vi "LSMHDR_write.vi"(8 "error in (no error)":errorcluster, 10 "LSMHDR":T1, 11 "refnum in":refnum<file>) -> (0 "error out":errorcluster, 3 "refnum out":refnum<file>)   [LabVIEW 2012]
uses:
  TTTR_data_headers/LSMHDR.ctl
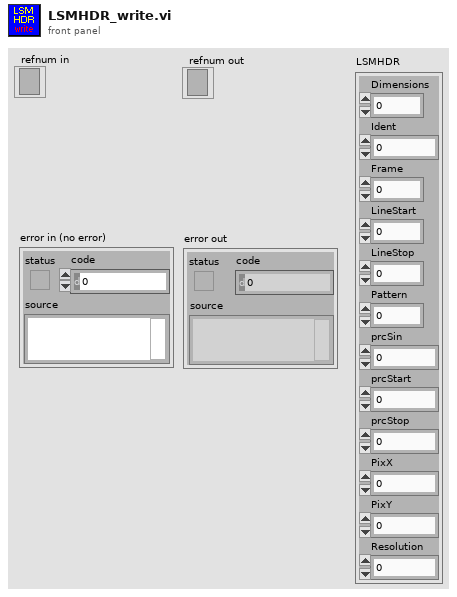
[diagram p1: front panel]
types:
  T1 = typedef "LSMHDR.ctl" = cluster{"Dimensions":i32, "Ident":i32, "Frame":i32, "LineStart":i32, "LineStop":i32, "Pattern":u8, "prcSin":u8, "prcStart":u8, "prcStop":u8, "PixX":i32, "PixY":i32, "Resolution":sgl}
  T2 = enum16{"big-endian, network order", "native, host order", "little-endian"}
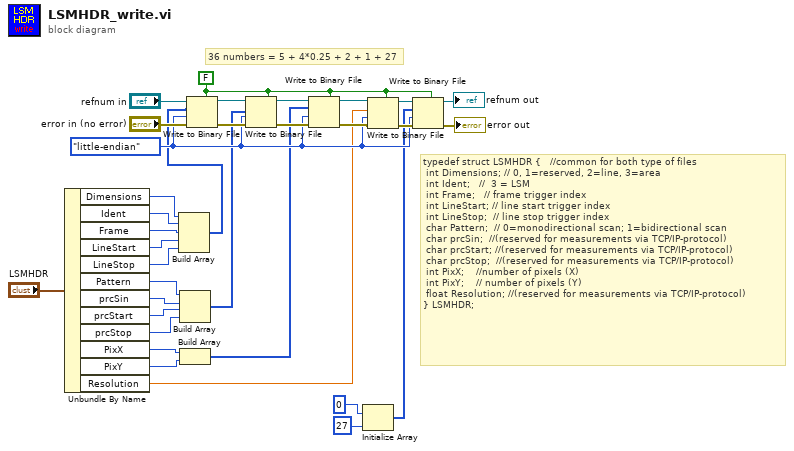
[diagram p0: block diagram]
diagram:
  w1 = FALSE ("prepend array or string size? (T)")
  w9 = T2."little-endian" ("byte order (0:big-endian, network order)")
  # "36 numbers = 5 + 4*0.25 + 2 + 1 + 27"
  # "typedef struct LSMHDR {\t\t\t//common for both type of files\n\tint Dimensions;\t// 0, 1=reserved, 2=line, 3=area\n\tint Ident;\t\t\t//  3 = LSM\n\tint Frame;\t\t\t// frame trigger index\n\tint LineStart;\t// line start trigger index\n\tint LineStop;\t\t// line stop trigger index\n char Pattern;\t\t// 0=monodirectional scan; 1=bidirectional scan\n\tchar prcSin;\t\t//(reserved for measurements via TCP/IP-protocol)\n\tchar prcStart;\t//(reserved for measurements via TCP/IP-protocol)\n\tchar prcStop;\t\t//(reserved for measurements via TCP/IP-protocol)\n\tint PixX;\t\t\t\t//number of pixels (X)\n\tint PixY;\t\t\t\t// number of pixels (Y)\n\tfloat Resolution;\t//(reserved for measurements via TCP/IP-protocol)\n} LSMHDR;"
  n1 = Unbundle By Name("LSMHDR") -> ("Dimensions"=w20:i32, "Ident"=w19:i32, "Frame"=w18:i32, "LineStart"=w17:i32, "LineStop"=w16:i32, "Pattern"=w15:u8, "prcSin"=w14:u8, "prcStart"=w13:u8, "prcStop"=w12:u8, "PixX"=w11:i32, "PixY"=w10:i32, "Resolution"=w5:sgl)
  n2 = Build Array(w20, w19, w18, w17, w16) -> (w8:i32[])
  n3 = Build Array(w15, w14, w13, w12) -> (w7:u8[])
  n4 = Build Array(w11, w10) -> (w6:i32[])
  n5 = Write to Binary File(file (use dialog)="refnum in", data=w8, error in="error in (no error)", 5:w1, 9:w9) -> (refnum out=w30:refnum<file>, error out=w31:errorcluster)  [unwired: 1 in, 1 out]
  n6 = Write to Binary File(file (use dialog)=w30, data=w7, error in=w31, 5:w1, 9:w9) -> (refnum out=w28:refnum<file>, error out=w29:errorcluster)  [unwired: 1 in, 1 out]
  n7 = Write to Binary File(file (use dialog)=w28, data=w6, error in=w29, 5:w1, 9:w9) -> (refnum out=w26:refnum<file>, error out=w27:errorcluster)  [unwired: 1 in, 1 out]
  n8 = Initialize Array(0, 27 ("count (1)")) -> (w2:i32[])
  n9 = Write to Binary File(file (use dialog)=w26, data=w5, error in=w27, 5:w1, 9:w9) -> (refnum out=w25:refnum<file>, error out=w23:errorcluster)  [unwired: 1 in, 1 out]
  n10 = Write to Binary File(file (use dialog)=w25, data=w2, error in=w23, 5:w1, 9:w9) -> (refnum out=→"refnum out":refnum<file>, error out=→"error out":errorcluster)  [unwired: 1 in, 1 out]
